vi "Delete Image.vi"(2 "Error":string, 3 "Image":T1={"Image ID"=0, "Channel ID"=-1}) -> (0 "Error":string)   [LabVIEW 2011, in "labvvis.lvlib"]
doc: "Deletes an existing image. Do not use the image after deletion."
uses:
  <userlib>/labvvis/labvvis.lvlib
  <userlib>/labvvis/VVIS Image.ctl
  labvvis.framework
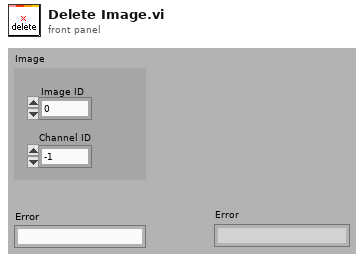
[diagram p1: front panel]
types:
  T1 = typedef "labvvis.lvlib/VVIS Image.ctl" = cluster{"Image ID":i16, "Channel ID":i16}
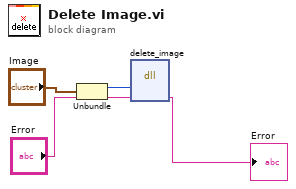
[diagram p0: block diagram]
diagram:
  n1 = Unbundle("Image") -> ("Image ID"=w3:i16)  [unwired: 1 out]
  n2 = dll-call lib="labvvis.framework" fn="delete_image"(w3, "error"="Error") -> ("error"=→"Error":string)  [unwired: 5 in, 2 out]
